vi "Filter Files by Extension.vi"(8 "error in (no error)":errorcluster, 10 "Extensions":string, 11 "Files":path[](array[path])) -> (0 "error out":errorcluster, 3 "Files out":path[](array[path]))   [LabVIEW 2020, in "VI Properties Editor.lvlib"]
doc: "Filters <B>Files</B> by <B>Extensions</B>."
uses:
  VI Properties Editor.lvlib
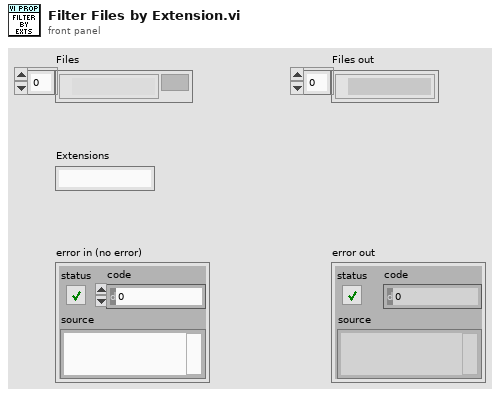
[diagram p1: front panel]
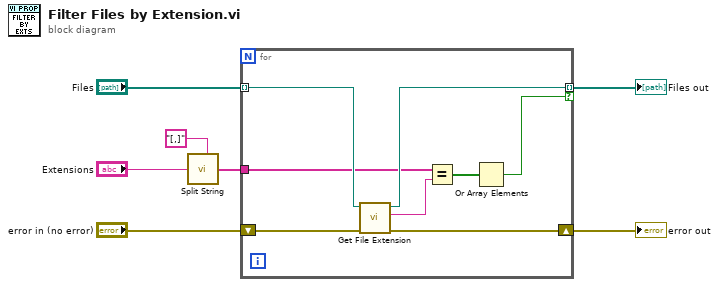
[diagram p0: block diagram]
diagram:
  n1 = call <vilib>:"Split String.vi"("Split Pattern"="[,]", "Input String"="Extensions") -> ("Split String"=w3:string[])  [unwired: 5 in]
  n2 = for {
    shift-right: [w14] -> w6
    shift-left: "error in (no error)" -> [w15]
    tunnel: w3 -> [w11]
    tunnel: "Files" -> [w13] mode=indexing
    tunnel: [w12] -> w1 mode=indexing if=w8
    n3 = call <vilib>:"Get File Extension.vi"("error in (no error)"=w15, "file"=w13) -> ("error out"=w14:errorcluster, "lowercase file extension"=w10:string, "dup file"=w12:path)  [unwired: 5 in, 2 out]
    n4 = Equal?(x=w11, y=w10) -> (x = y?=w9:bool[])
    n5 = Or Array Elements(Boolean array=w9) -> (logical OR=w8:bool)
  }
  "error out" <- w6
  "Files out" <- w1
